vi "Create Pattern Script - Write Frame.vi"(8 "error in (no error)":errorcluster, 11 "BML Pattern Creater in":refnum<class "BML Pattern Creater.lvclass">) -> (0 "error out":errorcluster, 2 "Script out":string, 3 "BML Pattern Creater out":refnum<class "BML Pattern Creater.lvclass">)   [LabVIEW 2018, in "BML Pattern Creater.lvlib" / "BML Pattern Creater.lvclass"]
uses:
  BML Pattern Creater.lvclass
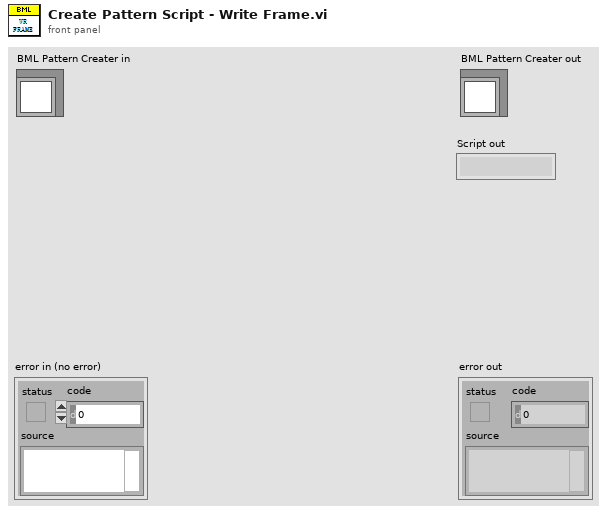
[diagram p1: front panel]
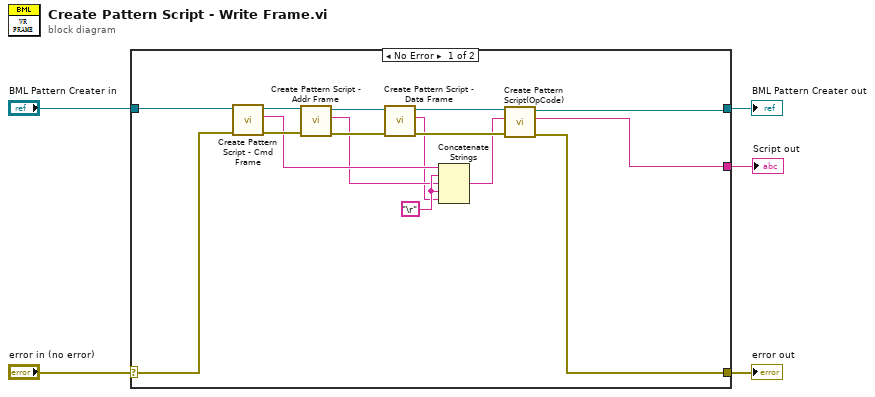
[diagram p0: block diagram]
diagram:
  n1 = case shown="No Error" "error in (no error)" {
    selector: "error in (no error)" -> [w18 w23]
    tunnel: [w6 w23] -> w4
    tunnel: [w7 w22] -> w2
    tunnel: "BML Pattern Creater in" -> [w20 w22]
    tunnel: [w8 _] -> w1
    frame No Error {
      w21 = "\r"
      n2 = call "Create Pattern Script - Cmd Frame.vi"("error in (no error)"=w18, "BML Pattern Creater in"=w20) -> ("error out"=w17:errorcluster, "CMD Frame out"=w12:string, "BML Pattern Creater out"=w19:refnum<class "BML Pattern Creater.lvclass">)  [unwired: 7 in]
      n3 = call "Create Pattern Script - Addr Frame.vi"("error in (no error)"=w17, "BML Pattern Creater in"=w19) -> ("error out"=w15:errorcluster, "Addr Frame"=w11:string, "BML Pattern Creater out"=w16:refnum<class "BML Pattern Creater.lvclass">)  [unwired: 7 in]
      n4 = call "Create Pattern Script - Data Frame.vi"("error in (no error)"=w15, "BML Pattern Creater in"=w16) -> ("error out"=w13:errorcluster, "Data Frame"=w10:string, "BML Pattern Creater out"=w14:refnum<class "BML Pattern Creater.lvclass">)  [unwired: 7 in]
      n5 = Concatenate Strings(w12, w21, w11, w21, w10) -> (w9:string)
      n6 = call "Create Pattern Script(OpCode).vi"("error in (no error)"=w13, "Write Script in"=w9, "BML Pattern Creater in"=w14) -> ("error out"=w6:errorcluster, "Script out"=w8:string, "BML Pattern Creater out"=w7:refnum<class "BML Pattern Creater.lvclass">)  [unwired: 6 in]
    }
    frame Error {
    }
  }
  "error out" <- w4
  "BML Pattern Creater out" <- w2
  "Script out" <- w1
